vi "Structure évènement.vi"() -> ()   [LabVIEW 2014]
panel:
  in  "stop":bool
  out "Choix":string
  in  "Bip":bool
  in  "Bonjour":bool
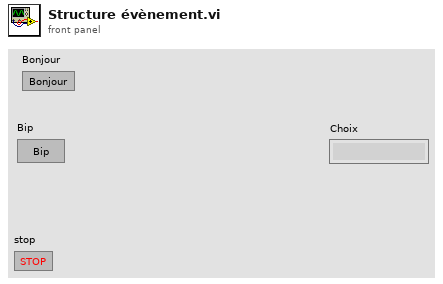
[diagram p1: front panel]
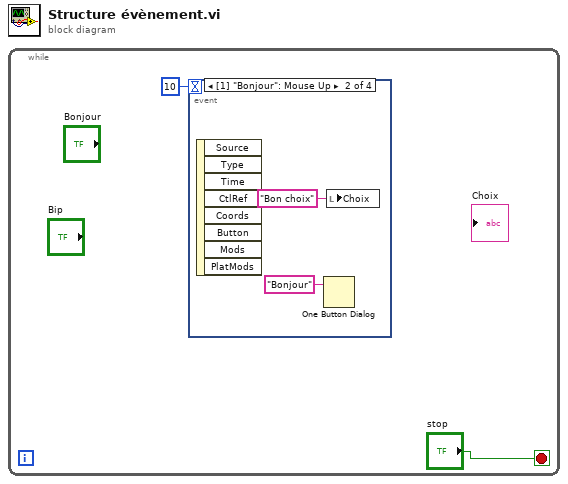
[diagram p0: block diagram]
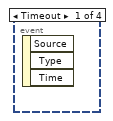
[diagram p2: hidden frame]
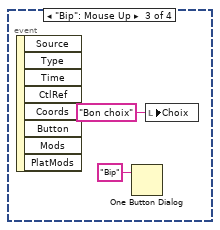
[diagram p3: hidden frame]
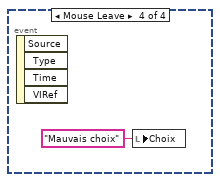
[diagram p4: hidden frame]
diagram:
  n1 = while {
    stop <- "stop" stop-if-true
    n2 = event shown="[1] \"Bonjour\": Mouse Up" {
      selector: _ -> [_ _ _ _]
      dyn-events: _ -> [_ _ _ _]
      timeout: 10 -> [_ _ _ _]
      event Timeout {
        n3 = event-data() -> ()  [unwired: 1 in, 3 out]
      }
      event "Bonjour": Mouse Up {
        n4 = event-data() -> ()  [unwired: 1 in, 8 out]
        n5 = One Button Dialog(message="Bonjour") -> ()  [unwired: 1 in, 1 out]
        n6 = local write "Choix"("Bon choix" ("Choix")) -> ()
      }
      event "Bip": Mouse Up {
        n7 = event-data() -> ()  [unwired: 1 in, 8 out]
        n8 = One Button Dialog(message="Bip") -> ()  [unwired: 1 in, 1 out]
        n9 = local write "Choix"("Bon choix" ("Choix")) -> ()
      }
      event Mouse Leave {
        n10 = event-data() -> ()  [unwired: 1 in, 4 out]
        n11 = local write "Choix"("Mauvais choix" ("result")) -> ()
      }
    }
  }
